vi "step6 FindStartingCorner.vi"(11 "cube in":T1) -> (2 "found start corner?":bool, 3 "cube out":T1)   [LabVIEW 2011]
uses:
  Typedef/cube.ctl
  Typedef/face.ctl
  Typedef/cube rotate direction.ctl
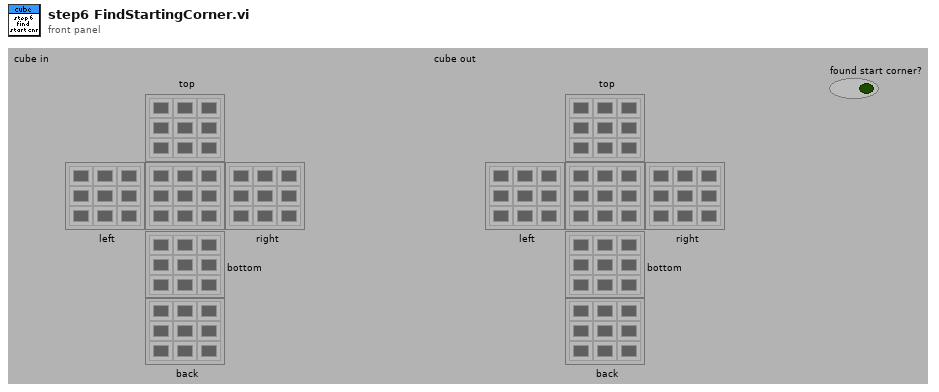
[diagram p1: front panel]
types:
  T1 = typedef "cube.ctl" = cluster{"top":T2, "left":T2, "right":T2, "bottom":T2, "back":T2, "front":T2}
  T2 = typedef "face.ctl" = u32[][]
  T3 = typedef "cube rotate direction.ctl" = enum16{"up", "down", "left", "right"}
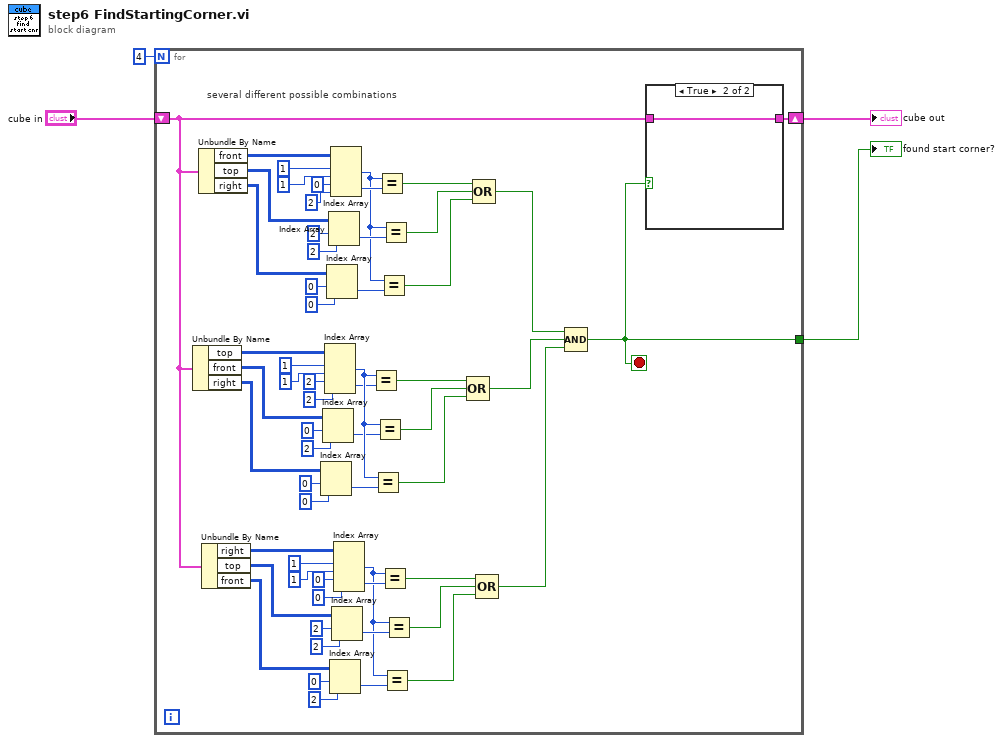
[diagram p0: block diagram]
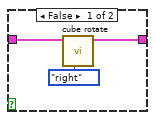
[diagram p2: hidden frame]
diagram:
  n1 = for {
    N: 4 -> [_]
    shift-right: [w62] -> w4
    shift-left: "cube in" -> [w9]
    tunnel: [w5] -> w3
    stop <- w5 stop-if-true
    # "several different possible combinations"
    n2 = Unbundle By Name(w9) -> ("top"=w30:T2, "front"=w34:T2, "right"=w41:T2)
    n3 = Unbundle By Name(w9) -> ("front"=w61:T2, "top"=w57:T2, "right"=w50:T2)
    n4 = Unbundle By Name(w9) -> ("right"=w25:T2, "top"=w21:T2, "front"=w14:T2)
    n5 = Index Array(array=w41, index (row)=0, index (col)=0 ("disabled index (col)")) -> (element=w38:u32)
    n6 = Index Array(array=w34, index (row)=0, index (col)=2 ("disabled index (col)")) -> (element=w37:u32)
    n7 = Index Array(array=w30, index (row) #1=1 ("index (row)"), index (col) #1=1 ("disabled index (col)"), index (row) #2=2 ("index (row)"), index (col) #2=2 ("disabled index (col)")) -> (element #1=w42:u32, element #2=w33:u32)
    n8 = Index Array(array=w50, index (row)=0, index (col)=0 ("disabled index (col)")) -> (element=w53:u32)
    n9 = Index Array(array=w57, index (row)=2, index (col)=2 ("disabled index (col)")) -> (element=w54:u32)
    n10 = Index Array(array=w14, index (row)=0, index (col)=2 ("disabled index (col)")) -> (element=w17:u32)
    n11 = Index Array(array=w61, index (row) #1=1 ("index (row)"), index (col) #1=1 ("disabled index (col)"), index (row) #2=0 ("index (row)"), index (col) #2=2 ("disabled index (col)")) -> (element #1=w49:u32, element #2=w58:u32)
    n12 = Index Array(array=w21, index (row)=2, index (col)=2 ("disabled index (col)")) -> (element=w18:u32)
    n13 = Index Array(array=w25, index (row) #1=1 ("index (row)"), index (col) #1=1 ("disabled index (col)"), index (row) #2=0 ("index (row)"), index (col) #2=0 ("disabled index (col)")) -> (element #1=w13:u32, element #2=w22:u32)
    n14 = Equal?(x=w42, y=w33) -> (x = y?=w43:bool)
    n15 = Equal?(x=w42, y=w38) -> (x = y?=w45:bool)
    n16 = Equal?(x=w42, y=w37) -> (x = y?=w44:bool)
    n17 = Equal?(x=w49, y=w58) -> (x = y?=w48:bool)
    n18 = Equal?(x=w49, y=w53) -> (x = y?=w46:bool)
    n19 = Equal?(x=w13, y=w22) -> (x = y?=w12:bool)
    n20 = Equal?(x=w49, y=w54) -> (x = y?=w47:bool)
    n21 = Equal?(x=w13, y=w17) -> (x = y?=w10:bool)
    n22 = Equal?(x=w13, y=w18) -> (x = y?=w11:bool)
    n23 = Compound Arithmetic op=OR(w43, w44, w45) -> (w7:bool)
    n24 = Compound Arithmetic op=OR(w48, w47, w46) -> (w8:bool)
    n25 = Compound Arithmetic op=OR(w12, w11, w10) -> (w6:bool)
    n26 = Compound Arithmetic op=AND(w8, w7, w6) -> (w5:bool)
    n27 = case shown="True" w5 {
      tunnel: w9 -> [w67 w68]
      tunnel: [w65 w68] -> w62
      frame False {
        n28 = call "cube rotate.vi"("cube rotation direction"=cube_rotate_direction."right", "cube in"=w67) -> ("cube out"=w65:T1)  [unwired: 8 in, 1 out]
      }
      frame True {
      }
    }
  }
  "cube out" <- w4
  "found start corner?" <- w3
